vi "MotorControllerV2.vi"(6 "Enable":bool, 8 "error in":errorcluster, 9 "Robot Velocities":T1 {"Angular Velocity (rad/s)" min=-1.0 max=1.0 scale=1.0..-1.0; "Y Velocity (m/s)" min=-1.0 max=1.0 scale=-1.0..1.0; "X Velocity (m/s)" min=-1.0 max=1.0 scale=-1.0..1.0}, 10 "FPGA VI Reference In":refnum<k20>, 11 "mecanum steering frame in":refnum<class "NI_Robotics_Mecanum Steering Frame.lvclass">) -> (0 "error out":errorcluster, 3 "steering frame out":refnum<class "NI_Robotics_Mecanum Steering Frame.lvclass">)   [LabVIEW 2012]
uses:
  <vilib>/robotics/Steering/Mecanum Steering Frame/NI_Robotics_Mecanum Steering Frame.lvclass
  <vilib>/robotics/Steering/Steering Frame/Apply Steering Frame Velocity to Motors.vi
  <vilib>/Utility/error.llb/Error Cluster From Error Code.vi
  <vilib>/rvi/errors/niLvFpgaAdjustHostInterfaceError.vi
  <vilib>/rvi/interface/nirviReadWriteControl/nirviReadWriteControl.xnode
  NiFpgaLv.dll
  <vilib>/rvi/interface/Simulation/niFpgaSimulationCallBeginRW.vi
  <vilib>/robotics/Steering/Steering Frame/NI_Robotics_Steering Frame.lvclass
panel:
  out "Front Left":dbl format="%#.2g"
  out "Front Right":dbl format="%#.2g"
  out "Rear Left":dbl format="%#.2g"
  out "Rear Right":dbl format="%#.2g"
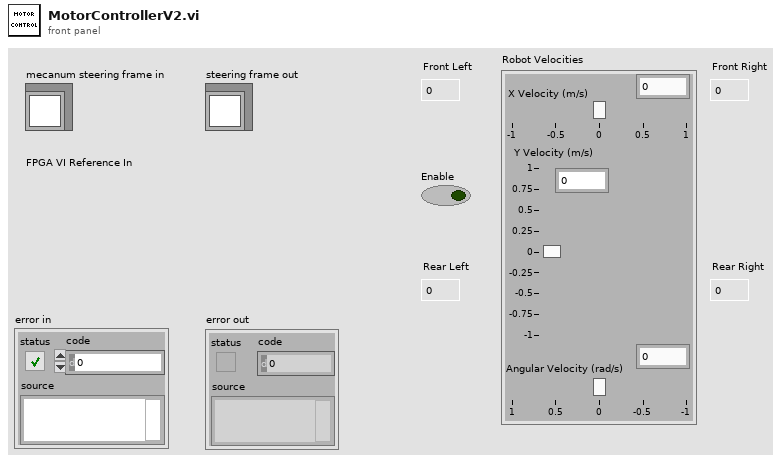
[diagram p1: front panel]
types:
  T1 = cluster{"X Velocity (m/s)":dbl, "Y Velocity (m/s)":dbl, "Angular Velocity (rad/s)":dbl}
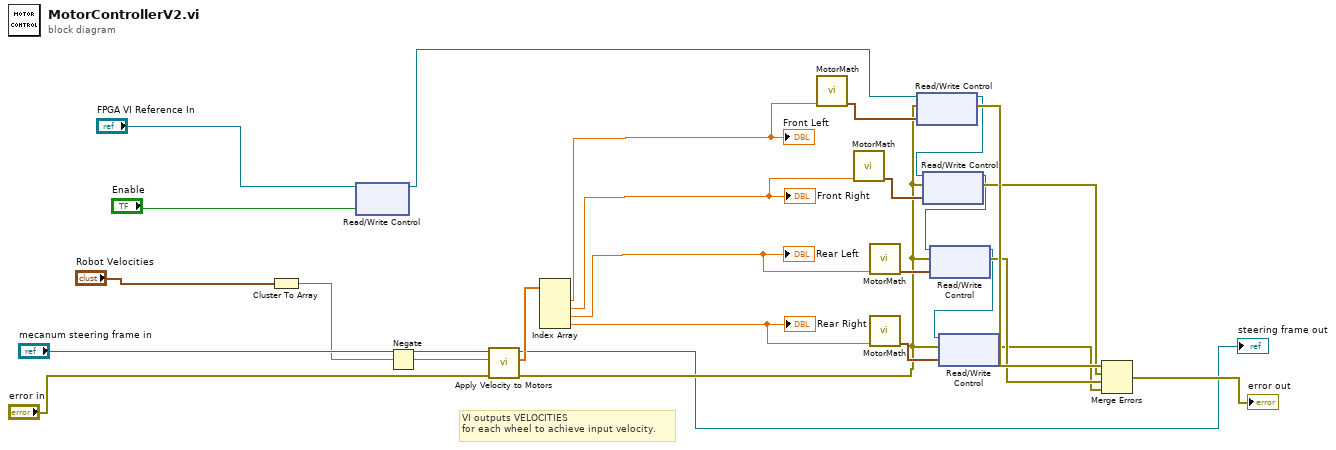
[diagram p0: block diagram]
diagram:
  # "VI outputs VELOCITIES\nfor each wheel to achieve input velocity."
  n1 = Cluster To Array(cluster="Robot Velocities") -> (array=w3:dbl[])
  n2 = xnode "Read/Write Control"("FPGA VI Reference In"="FPGA VI Reference In", "Enable"="Enable") -> ("FPGA VI Reference Out"=w2:refnum<k20>)  [unwired: 1 in, 1 out]
  n3 = Negate(x=w3) -> (-x=w1:dbl[])
  n4 = call-poly <vilib>:"Apply Velocity to Motors.vi"("error in (no error)"="error in", "steering frame velocity"=w1, "steering frame in"="mecanum steering frame in") -> ("error out"=w10:errorcluster, "ccw motor velocity setpoints"=w15:dbl[], "steering frame out"=→"steering frame out":refnum<class "NI_Robotics_Mecanum Steering Frame.lvclass">)  [unwired: 4 in, 2 out]
  n5 = Index Array(array=w15) -> (element #1=w11:dbl, element #2=w12:dbl, element #3=w13:dbl, element #4=w14:dbl)  [unwired: 4 in]
  "Front Left" <- w11
  "Front Right" <- w12
  "Rear Left" <- w13
  "Rear Right" <- w14
  n6 = call "MotorMath.vi"("Motor velocity"=w11) -> ("output cluster"=w27:cluster{i32, "upper limit":dbl})  [unwired: 10 in]
  n7 = call "MotorMath.vi"("Motor velocity"=w12) -> ("output cluster"=w26:cluster{i32, "upper limit":dbl})  [unwired: 10 in]
  n8 = call "MotorMath.vi"("Motor velocity"=w13) -> ("output cluster"=w25:cluster{i32, "upper limit":dbl})  [unwired: 10 in]
  n9 = call "MotorMath.vi"("Motor velocity"=w14) -> ("output cluster"=w24:cluster{i32, "upper limit":dbl})  [unwired: 10 in]
  n10 = xnode "Read/Write Control"("FPGA VI Reference In"=w2, "error in"=w10, "Motor 1"=w27) -> ("FPGA VI Reference Out"=w18:refnum<k20>, "error out"=w23:errorcluster)
  n11 = xnode "Read/Write Control"("FPGA VI Reference In"=w18, "error in"=w10, "Motor 2"=w26) -> ("FPGA VI Reference Out"=w17:refnum<k20>, "error out"=w22:errorcluster)
  n12 = xnode "Read/Write Control"("FPGA VI Reference In"=w17, "error in"=w10, "Motor 3"=w25) -> ("FPGA VI Reference Out"=w16:refnum<k20>, "error out"=w21:errorcluster)
  n13 = xnode "Read/Write Control"("FPGA VI Reference In"=w16, "error in"=w10, "Motor 4"=w24) -> ("error out"=w20:errorcluster)  [unwired: 1 out]
  n14 = Merge Errors(w23, w22, w21, w20) -> (→"error out":errorcluster)
